vi "电压-电量.vi"(11 "输出电压":dbl) -> (3 "电量":dbl)   [LabVIEW 2018]
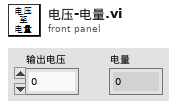
[diagram p1: front panel]
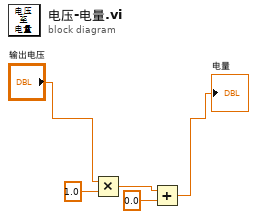
[diagram p0: block diagram]
diagram:
  n1 = Multiply(x="输出电压", y=1.0) -> (x*y=w3:dbl)
  n2 = Add(x=w3, y=0.0) -> (x+y=→"电量":dbl)
